vi "SMO.Dictionary.GetKeys.vi"(6 "timeout (10ms)":i32=10, 8 "error in (no error)":errorcluster, 11 "SMO.Dictionary":refnum<class "SMO.Dictionary.lvclass">) -> (0 "error out":errorcluster, 2 "Keys":string[](array[string]), 3 "SMO.Dictionary out":refnum<class "SMO.Dictionary.lvclass">, 4 "timed out?":bool)   [LabVIEW 2013, in "SMO.Dictionary.lvlib" / "SMO.Dictionary.lvclass"]
doc: "---------------------------------------------------------------\nJKI State Machine Objects™\nhttp://jki.net/state-machine-objects/\nCopyright (C) 2005-2015, JKI <info@jki.net>\nALL RIGHTS RESERVEDJKI State Machine Objects (SMO) 1.0.0.4\nJKI - JKI\nCopyright (c) 2015, JKI"
uses:
  SMO.Dictionary.lvclass
panel:
  # "For instructions on how to use the JKI State Machine Objects, examples and video tutorials, visit:\nhttp://jki.net/state-machine-objects/\n\nJKI State Machine Objects™\nhttp://jki.net/state-machine-objects/\nCopyright (C) 2005-2015, JKI <info@jki.net>\nALL RIGHTS RESERVED"
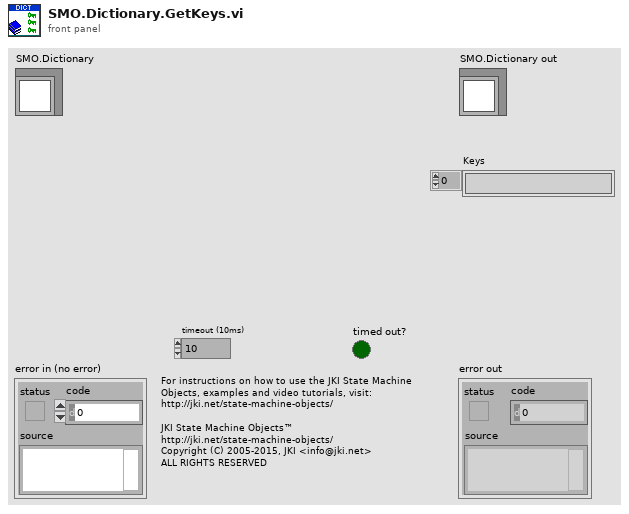
[diagram p1: front panel]
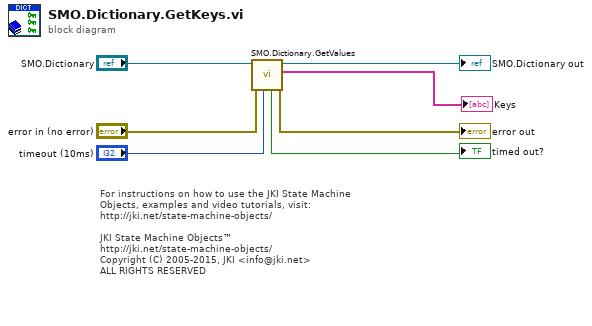
[diagram p0: block diagram]
diagram:
  # "For instructions on how to use the JKI State Machine Objects, examples and video tutorials, visit:\nhttp://jki.net/state-machine-objects/\n\nJKI State Machine Objects™\nhttp://jki.net/state-machine-objects/\nCopyright (C) 2005-2015, JKI <info@jki.net>\nALL RIGHTS RESERVED"
  n1 = call "SMO.Dictionary.GetValues.vi"("timeout (10ms)"="timeout (10ms)", "error in (no error)"="error in (no error)", "SMO.Dictionary"="SMO.Dictionary") -> ("error out"=→"error out":errorcluster, "Keys out"=→"Keys":string[], "SMO.Dictionary out"=→"SMO.Dictionary out":refnum<class "SMO.Dictionary.lvclass">, "timed out?"=→"timed out?":bool)  [unwired: 4 in, 1 out]
